vi "Open Acrobat Document.vi"(4 "error in (no error)":errorcluster, 7 "acrobat document":path) -> (0 "error out":errorcluster)   [LabVIEW 2015]
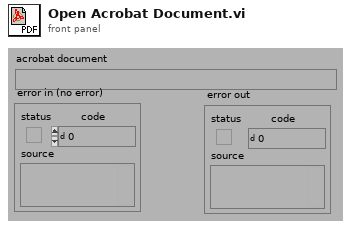
[diagram p1: front panel]
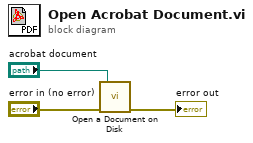
[diagram p0: block diagram]
diagram:
  n1 = call "Open a Document on Disk.vi"("error in (no error)"="error in (no error)", "document path"="acrobat document") -> ("error out"=→"error out":errorcluster)  [unwired: 5 in]
